vi "Main.vi"() -> ()   [LabVIEW 2017]
panel:
  out "Output":string
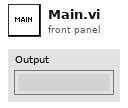
[diagram p1: front panel]
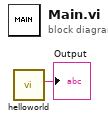
[diagram p0: block diagram]
diagram:
  n1 = call "helloworld.vi"() -> ("Output/Failure"=→"Output":string)  [unwired: 10 in, 1 out]
